vi "TCP-Send String (byte array).vi"(0 "PXI Address":string, 5 "Port":i32, 7 "string":string, 9 "timeout (ms)":i32=5000, 11 "error in (no error)":errorcluster) -> (8 "result":i32, 15 "error out":errorcluster)   [LabVIEW 2020]
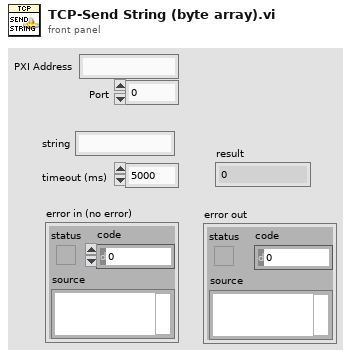
[diagram p1: front panel]
types:
  T1 = enum16{"Standard", "Buffered", "CRLF", "Immediate"}
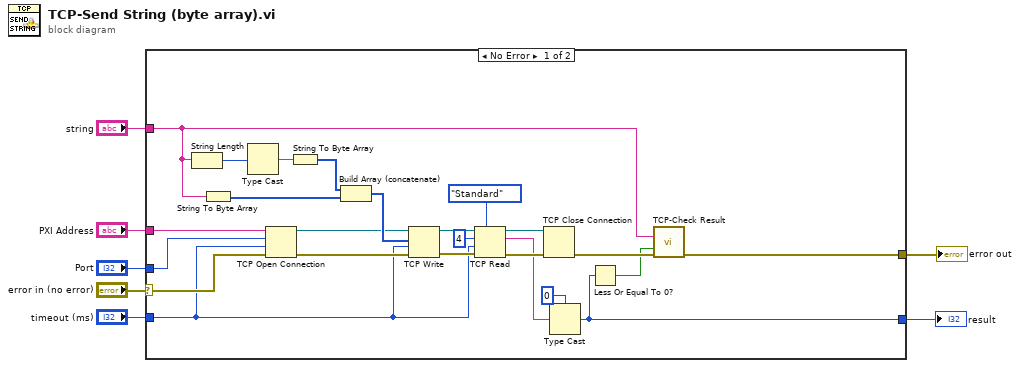
[diagram p0: block diagram]
diagram:
  n1 = case shown="No Error" "error in (no error)" {
    selector: "error in (no error)" -> [w26 w32]
    tunnel: "Port" -> [w29 _]
    tunnel: "PXI Address" -> [w28 _]
    tunnel: [w25 _] -> w4
    tunnel: [w10 w32] -> w3
    tunnel: "timeout (ms)" -> [w15 _]
    tunnel: "string" -> [w9 _]
    frame No Error {
      n2 = String Length(string=w9) -> (length=w14:i32)
      n3 = String To Byte Array(string=w9) -> (unsigned byte array=w31:u8[])
      n4 = Type Cast(x=w14) -> (*(type *) &x=w13:string)  [unwired: 1 in]
      n5 = TCP Open Connection(address=w28, remote port or service name=w29, timeout ms (60000)=w15, error in (no error)=w26) -> (connection ID=w27:refnum<k5>, error out=w16:errorcluster)  [unwired: 1 in]
      n6 = String To Byte Array(string=w13) -> (unsigned byte array=w12:u8[])
      n7 = Build Array (concatenate)(w12, w31) -> (w30:u8[])
      n8 = TCP Write(connection ID=w27, data in=w30, error in (no error)=w16, 9:w15) -> (connection ID out=w18:refnum<k5>, error out=w17:errorcluster)  [unwired: 1 out]
      n9 = TCP Read(connection ID=w18, bytes to read=4, error in (no error)=w17, 7:T1."Standard" ("mode (standard)"), 9:w15) -> (connection ID out=w19:refnum<k5>, data out=w20:string, error out=w24:errorcluster)
      n10 = TCP Close Connection(connection ID=w19, error in (no error)=w24) -> (error out=w11:errorcluster)  [unwired: 1 in, 1 out]
      n11 = Type Cast(type=0, x=w20) -> (*(type *) &x=w25:i32)
      n12 = Less Or Equal To 0?(x=w25) -> (x <= 0?=w8:bool)
      n13 = call "TCP-Check Result.vi"("command"=w9, "invalid response"=w8, "error IO"=w11) -> ("error out"=w10:errorcluster)  [unwired: 12 in]
    }
    frame Error {
    }
  }
  "error out" <- w3
  "result" <- w4
